vi "Main2.vi"() -> ()   [LabVIEW 2019]
uses:
  <vilib>/myRIO/Instrument Drivers/Utilities/Utilities.lvlib
panel:
  in  "Motor 4":dbl
  in  "Motor 3":dbl
  in  "Motor 2":dbl
  in  "Motor 1":dbl
  in  "error in (no error)":errorcluster
  out "error out":errorcluster
  out "error out 2":errorcluster
  out "error out 3":errorcluster
  out "error out 4":errorcluster
  out "error out 5":errorcluster
  out "error out 6":errorcluster
  in  "PID Gains":T1={"Proportional Gain (Kc)"=0.8, "Integral Gain"=25.0, "Derivative Gain"=0.004}
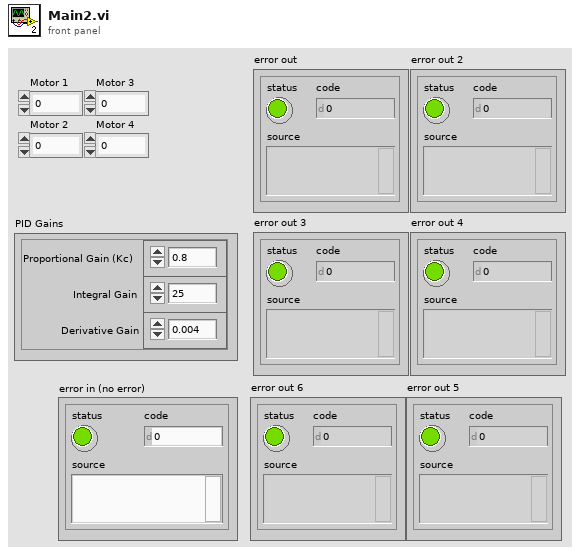
[diagram p1: front panel]
types:
  T1 = cluster{"Proportional Gain (Kc)":dbl, "Integral Gain":dbl, "Derivative Gain":dbl}
  T2 = cluster{"[0]":dbl, "[1]":dbl, "[2]":dbl, "[3]":dbl, "[4]":dbl, "[5]":dbl, "[6]":dbl, "[7]":dbl, "[8]":dbl}
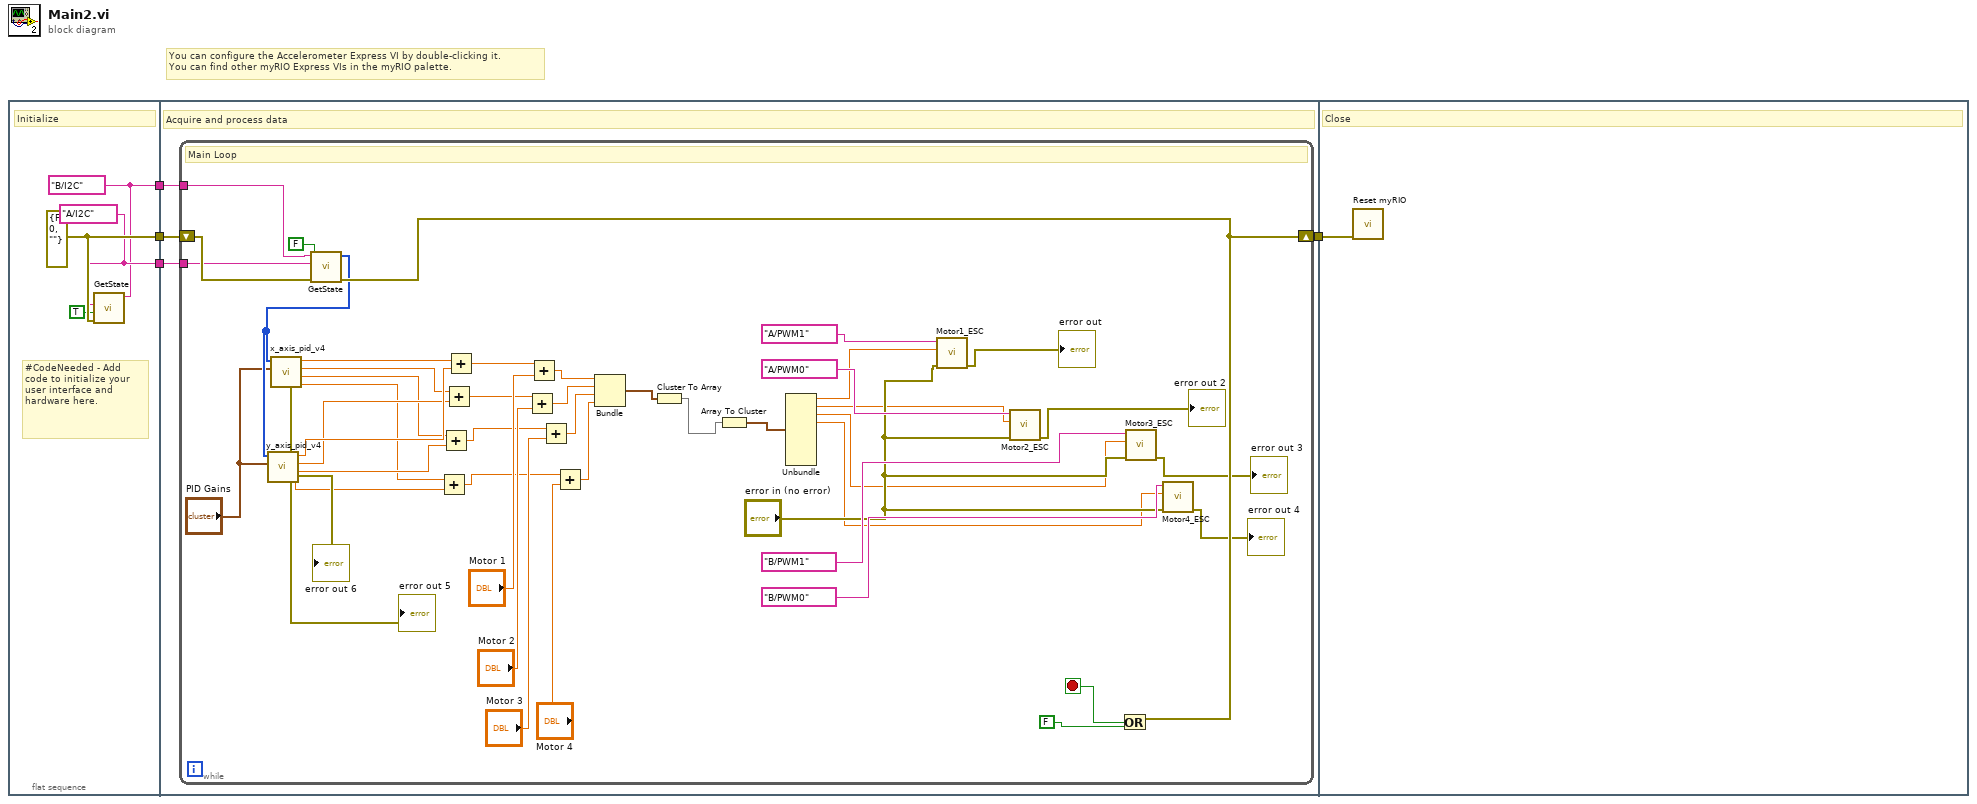
[diagram p0: block diagram]
diagram:
  # "You can configure the Accelerometer Express VI by double-clicking it.\nYou can find other myRIO Express VIs in the myRIO palette."
  n1 = flat-sequence {
    tunnel: [w8] -> w4
    tunnel: [w6] -> w3
    tunnel: [w7] -> w2
    tunnel: w4 -> [w12]
    tunnel: [w11] -> w1
    tunnel: w3 -> [w10]
    tunnel: w2 -> [w9]
    tunnel: w1 -> [w60]
    frame #0 {
      w7 = tag "A/I2C" ("IMU Channel")
      w6 = tag "B/I2C" ("LIDAR Channel")
      w8 = errorcluster {"status"=FALSE, "code"=0, "source"=""} ("error in (no error)")
      # "#CodeNeeded - Add code to initialize your user interface and hardware here."
      # "Initialize"
      n2 = call "GetState.vi"("error in (no error)"=w8, "Calibrate?"=TRUE, "IMU Channel"=w7, "LIDAR Channel"=w6) -> ()  [unwired: 2 in, 4 out]
    }
    frame #1 {
      # "Acquire and process data"
      n3 = while {
        shift-right: [w54] -> w11
        shift-left: w12 -> [w58]
        tunnel: w10 -> [w56]
        tunnel: w9 -> [w55]
        stop <- w59 stop-if-true
        # "Main Loop"
        n4 = call "GetState.vi"("error in (no error)"=w58, "Calibrate?"=FALSE, "IMU Channel"=w55, "LIDAR Channel"=w56) -> ("error out"=w54:errorcluster, "imu accel"=w41:i16[])  [unwired: 2 in, 2 out]
        n5 = call "y_axis_pid_v4.vi"("PID Gains"="PID Gains", "Y In"=w41) -> ("Motor 4"=w33:dbl, "Motor 3"=w35:dbl, "Motor 2"=w36:dbl, "Motor 1"=w38:dbl, "error out"=→"error out 6":errorcluster)  [unwired: 5 in]
        n6 = call "x_axis_pid_v4.vi"("PID Gains"="PID Gains", "X In"=w41) -> ("Motor 4"=w34:dbl, "Motor 3"=w32:dbl, "Motor 2"=w37:dbl, "Motor 1"=w39:dbl, "error out"=→"error out 5":errorcluster)  [unwired: 5 in]
        n7 = Add(x=w34, y=w33) -> (x+y=w21:dbl)
        n8 = Add(x=w32, y=w35) -> (x+y=w20:dbl)
        n9 = Add(x=w37, y=w36) -> (x+y=w19:dbl)
        n10 = Add(x=w39, y=w38) -> (x+y=w25:dbl)
        n11 = Add(x=w19, y="Motor 2") -> (x+y=w17:dbl)
        n12 = Add(x=w25, y="Motor 1") -> (x+y=w18:dbl)
        n13 = Add(x=w20, y="Motor 3") -> (x+y=w16:dbl)
        n14 = Add(x=w21, y="Motor 4") -> (x+y=w15:dbl)
        n15 = Bundle(w18, w17, w16, w15) -> (w14:cluster{dbl, dbl, dbl, dbl})  [unwired: 1 in]
        n16 = Cluster To Array(cluster=w14) -> (array=w13:dbl[])
        n17 = Array To Cluster(array=w13) -> (cluster=w27:T2)
        n18 = Unbundle(w27) -> ("[0]"=w31:dbl, "[1]"=w30:dbl, "[2]"=w29:dbl, "[3]"=w28:dbl)  [unwired: 5 out]
        n19 = call "Motor1_ESC.vi"("error in (no error)"="error in (no error)", "Percent Power"=w31, "Channel Name"=tag "A/PWM1") -> ("error out"=→"error out":errorcluster)  [unwired: 8 in]
        n20 = call "Motor2_ESC.vi"("error in (no error)"="error in (no error)", "Percent Power"=w30, "Channel Name"=tag "A/PWM0") -> ("error out"=→"error out 2":errorcluster)  [unwired: 8 in]
        n21 = Or(x=w54, y=FALSE) -> (x .or. y?=w59:bool)
        n22 = call "Motor3_ESC.vi"("error in (no error)"="error in (no error)", "Percent Power"=w29, "Channel Name"=tag "B/PWM1") -> ("error out"=→"error out 3":errorcluster)  [unwired: 8 in]
        n23 = call "Motor4_ESC.vi"("error in (no error)"="error in (no error)", "Percent Power"=w28, "Channel Name"=tag "B/PWM0") -> ("error out"=→"error out 4":errorcluster)  [unwired: 8 in]
      }
    }
    frame #2 {
      # "Close"
      n24 = call <vilib>:"Reset myRIO.vi"("error in (no error)"=w60) -> ()  [unwired: 10 in, 1 out]
    }
  }
